vi "Get all info.vi"(8 "error in (no error)":errorcluster, 11 "VISA Refnum in":refnum<visa-resource-name>) -> (0 "error out":errorcluster, 2 "Recibo de Datos":string, 3 "VISA Refnum out":refnum<visa-resource-name>)   [LabVIEW 2025, in "Control de MaP.lvlib"]
uses:
  Control de MaP.lvlib
  Write--command.vi
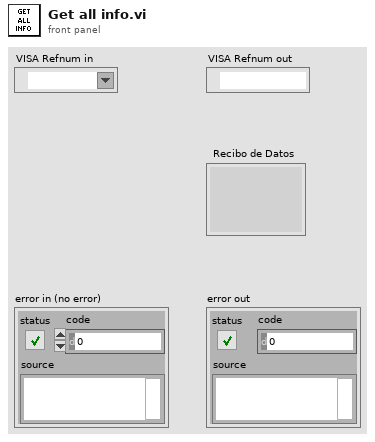
[diagram p1: front panel]
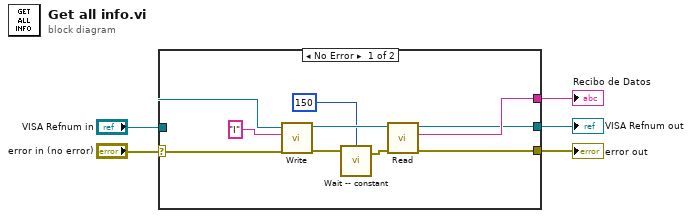
[diagram p0: block diagram]
diagram:
  n1 = case shown="No Error" "error in (no error)" {
    selector: "error in (no error)" -> [w11 w17]
    tunnel: [w15 _] -> w5
    tunnel: [w14 w16] -> w4
    tunnel: "VISA Refnum in" -> [w13 w16]
    tunnel: [w12 w17] -> w2
    frame No Error {
      n2 = call-poly "Write.vi"("error in (no error)"=w11, "Command"="I", "VISA resource name"=w13) -> ("error out"=w7:errorcluster, "VISA resource name out"=w9:refnum<visa-resource-name>)  [unwired: 6 in, 1 out]
      n3 = call "Wait -- constant.vi"("wait (200 ms)"=u32 150, "error in (no error)"=w7) -> ("error out"=w8:errorcluster)  [unwired: 3 in]
      n4 = call "Read.vi"("error in (no error)"=w8, "VISA resource name"=w9) -> ("error out"=w12:errorcluster, "Recibo de Datos"=w15:string, "VISA resource name out"=w14:refnum<visa-resource-name>)  [unwired: 6 in, 1 out]
    }
    frame Error {
    }
  }
  "Recibo de Datos" <- w5
  "VISA Refnum out" <- w4
  "error out" <- w2
